vi "SetParam.vi"(8 "error in (no error)":errorcluster, 10 "image_size":cluster{"image_height":i32, "image_width":i32}, 11 "Reconstruct_from_patches_2d in":refnum<class "Reconstruct_from_patches_2d.lvclass">) -> (0 "error out":errorcluster, 3 "Reconstruct_from_patches_2d out":refnum<class "Reconstruct_from_patches_2d.lvclass">)   [LabVIEW 2020, in "Reconstruct_from_patches_2d.lvclass"]
uses:
  Reconstruct_from_patches_2d.lvclass
  Reconstruct_from_patches_2d.lvclass/Reconstruct_from_patches_2d.ctl
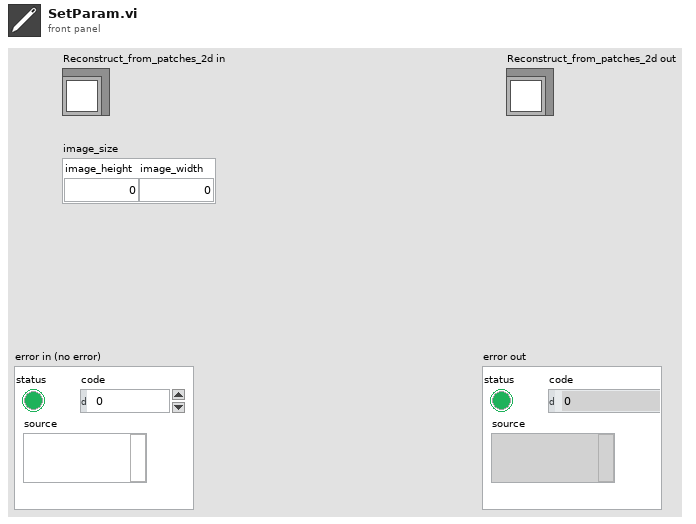
[diagram p1: front panel]
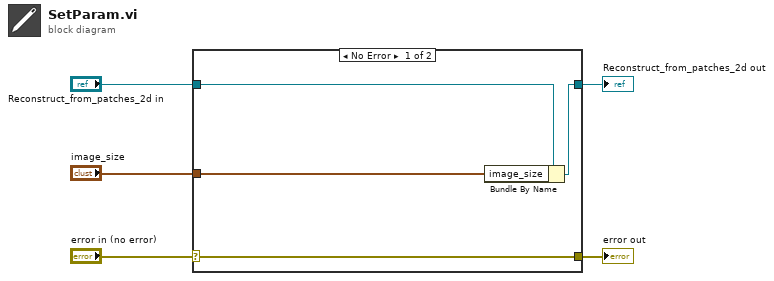
[diagram p0: block diagram]
diagram:
  n1 = case shown="No Error" "error in (no error)" {
    selector: "error in (no error)" -> [w9 w10]
    tunnel: [w9 w10] -> w4
    tunnel: [w7 w11] -> w2
    tunnel: "Reconstruct_from_patches_2d in" -> [w8 w11]
    tunnel: "image_size" -> [w6 _]
    frame No Error {
      n2 = Bundle By Name(cluster=w8, "image_size"=w6) -> (w7:refnum<class "Reconstruct_from_patches_2d.lvclass">)
    }
    frame Error {
    }
  }
  "error out" <- w4
  "Reconstruct_from_patches_2d out" <- w2
